vi "Thev-Show Progress Table.vi"(0 "Table in":refnum<vi>, 5 "progress":T1[](array[typedef])) -> ()   [LabVIEW 2015]
uses:
  Typedefs/Thev-Progress Table Element.ctl
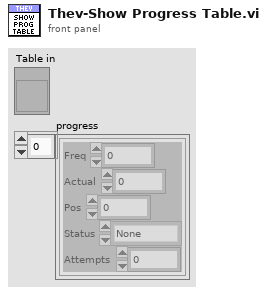
[diagram p1: front panel]
types:
  T1 = typedef "Thev-Progress Table Element.ctl" = cluster{"Freq":dbl, "Actual":dbl, "Pos":dbl, "Status":enum16{"None", "Measuring", "Finished"}, "Attempts":i32}
  T2 = enum16{"User", "Prism", "Kelly", "Dark2", "Sequential", "Hue"}
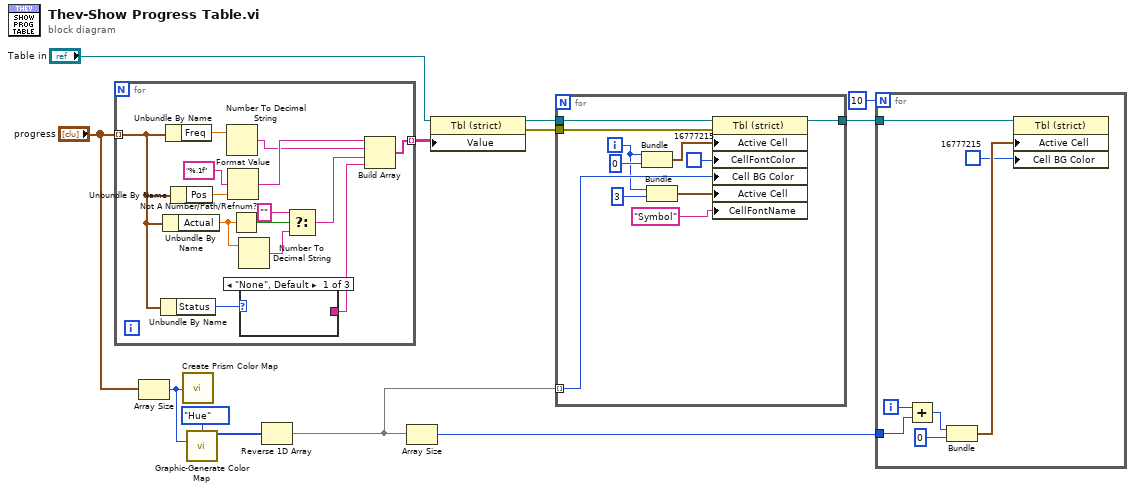
[diagram p0: block diagram]
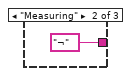
[diagram p2: hidden frame]
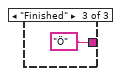
[diagram p3: hidden frame]
diagram:
  n1 = for {
    tunnel: "progress" -> [w17] mode=indexing
    tunnel: [w25] -> w12 mode=indexing
    n2 = Unbundle By Name(w17) -> ("Status"=w16:enum16{"None", "Measuring", "Finished"})
    n3 = Unbundle By Name(w17) -> ("Actual"=w22:dbl)
    n4 = Unbundle By Name(w17) -> ("Freq"=w26:dbl)
    n5 = Unbundle By Name(w17) -> ("Pos"=w24:dbl)
    n6 = Number To Decimal String(number=w26) -> (decimal integer string=w13:string)  [unwired: 1 in]
    n7 = Format Value(format string="%.1f", value (0)=w24) -> (output string=w14:string)  [unwired: 1 in]
    n8 = Not A Number/Path/Refnum?(number/path/refnum=w22) -> (NaN/Path/Refnum?=w20:bool)
    n9 = Number To Decimal String(number=w22) -> (decimal integer string=w21:string)  [unwired: 1 in]
    n10 = case shown="\"None\", Default" w16 {
      tunnel: [_ "¬" "Ö"] -> w15
      frame "None", Default {
      }
      frame "Measuring" {
      }
      frame "Finished" {
      }
    }
    n11 = Select(t="", s=w20, f=w21) -> (s? t:f=w18:string)
    n12 = Build Array(w14, w13, w18, w15) -> (w25:string[])
  }
  n13 = Array Size(array="progress") -> (size(s)=w6:i32)
  n14 = call "Create Prism Color Map.vi"("Size"=w6) -> ()  [unwired: 1 out]
  n15 = call "Graphic-Generate Color Map.vi"("Map"=T2."Hue", "Size"=w6) -> ("Colors"=w5:u32[])  [unwired: 13 in]
  n16 = Reverse 1D Array(array=w5) -> (reversed array=w2:u32[])
  n17 = Array Size(array=w2) -> (size(s)=w1:i32)
  n18 = property class="Tbl (strict)"(reference="Table in", "Value"=w12) -> (reference out=w9:refnum<vi>, error out=w8:errorcluster)  [unwired: 1 in]
  n19 = for {
    tunnel: w9 -> [w39]
    tunnel: w8 -> [w38]
    tunnel: w2 -> [w35] mode=indexing
    tunnel: [w29] -> w4
    i -> [w33]
    n20 = Bundle(w33, 0) -> (w36:cluster{i32, i32})  [unwired: 1 in]
    n21 = Bundle(w33, 3) -> (w31:cluster{i32, i32})  [unwired: 1 in]
    n22 = property class="Tbl (strict)"(reference=w39, error in=w38, "Active Cell"=w36, "CellFontColor"=u32 16777215, "Cell BG Color"=w35, "Active Cell"=w31, "CellFontName"="Symbol" ("Active Cell:Cell Font:Name")) -> (reference out=w29:refnum<vi>)  [unwired: 1 out]
  }
  n23 = for {
    N: 10 -> [_]
    tunnel: w4 -> [w46]
    tunnel: w1 -> [w44]
    i -> [w45]
    n24 = Add(x=w45, y=w44) -> (x+y=w42:i32)
    n25 = Bundle(w42, 0) -> (w41:cluster{i32, i32})  [unwired: 1 in]
    n26 = property class="Tbl (strict)"(reference=w46, "Active Cell"=w41, "Cell BG Color"=u32 16777215) -> ()  [unwired: 1 in, 2 out]
  }
